vi "CameraGetScaledAttrSharpness.vi"(8 "error in (no error)":errorcluster, 10 "Attr String":string, 11 "IMAQdx Session":T1) -> (0 "error out":errorcluster, 1 "Raw":dbl, 2 "Scaled":dbl, 3 "IMAQdx Session out":T1)   [LabVIEW 2023]
doc: "Returns the scaled and raw value of a numeric camera attribute.\n\n\nThis software is licensed. Open the labview\\readme\\WPI Robotics Library Open Source License.txt file for more information."
uses:
  <vilib>/userDefined/High Color/IMAQdx.ctl
  <resource>/objmgr/imaqdx.rc
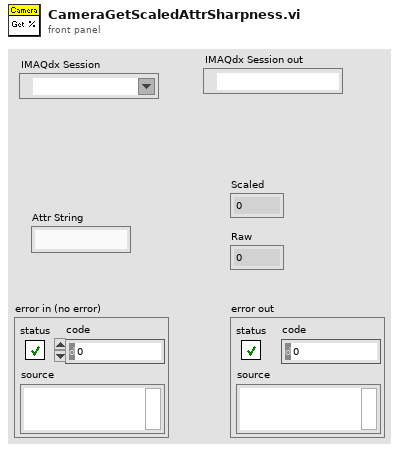
[diagram p1: front panel]
types:
  T1 = typedef "IMAQdx.ctl" = refnum<k21>
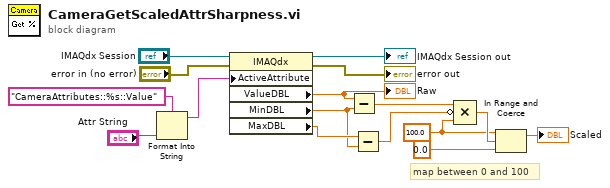
[diagram p0: block diagram]
diagram:
  w8 = 100.0
  # "map between 0 and 100"
  n1 = Format Into String(format string="CameraAttributes::%s::Value" ("Attr Format"), "Attr String") -> (resulting string=w15:string)  [unwired: 2 in, 1 out]
  n2 = property class="IMAQdx"(reference="IMAQdx Session", error in="error in (no error)", "ActiveAttribute"=w15) -> (reference out=→"IMAQdx Session out":T1, error out=→"error out":errorcluster, "ValueDBL"=w14:dbl, "MinDBL"=w12:dbl, "MaxDBL"=w13:dbl)
  "Raw" <- w14
  n3 = Subtract(x=w14, y=w12) -> (x-y=w11:dbl)
  n4 = Subtract(x=w13, y=w12) -> (x-y=w10:dbl)
  n5 = Compound Arithmetic op=MULTIPLY(w11, invert w10, w8) -> (w9:dbl)
  n6 = In Range and Coerce(upper limit=w8, x=w9, lower limit=0.0) -> (coerced(x)=→"Scaled":dbl)  [unwired: 1 out]
